vi "NR_LDPC_Decode_opti.vi"(0 "appended path":path, 1 "Zc":dbl, 2 "LDPC_base_graph":dbl, 5 "C":dbl, 9 "cdblkseg_data":dbl[][](array[numeric]), 11 "dermdata":dbl[][](array[numeric]), 12 "EN_LDPC":dbl, 14 "error in (no error)":errorcluster caption="错误输入（无错误）") -> (3 "deldpccode":dbl[][](array[numeric]), 15 "error IO":errorcluster)   [LabVIEW 2015]
panel:
  in  "H":dbl[][](array[numeric])
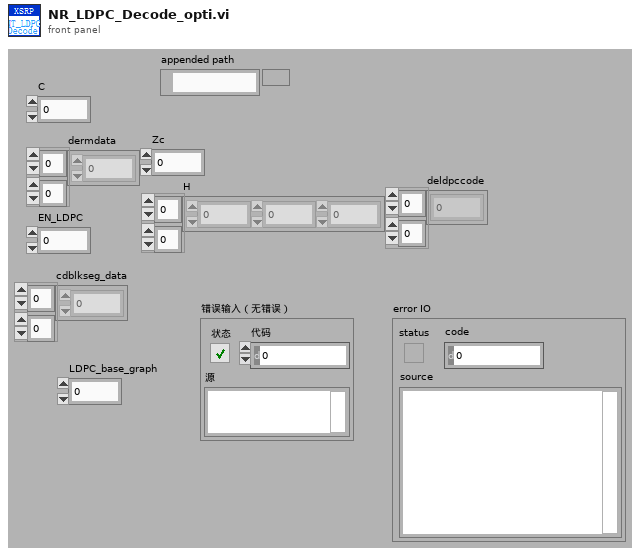
[diagram p1: front panel]
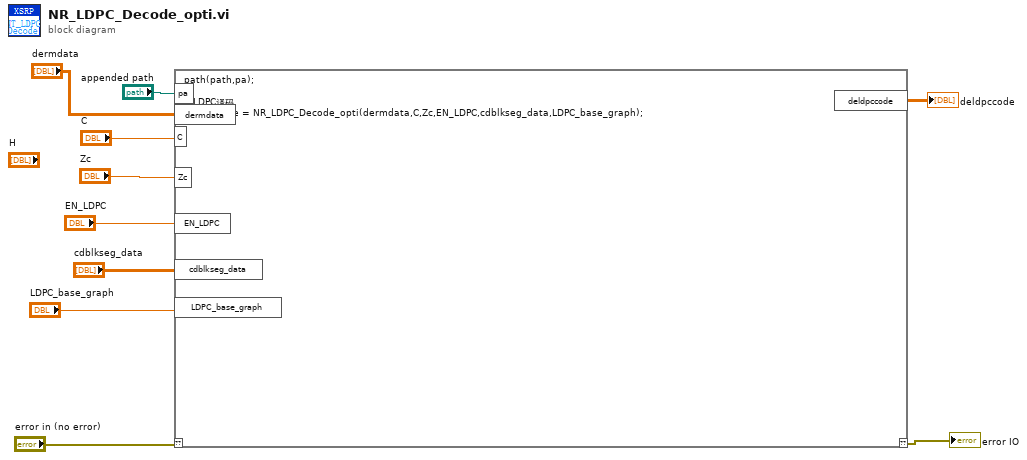
[diagram p0: block diagram]
diagram:
  n1 = script code="path(path,pa);\n\n%LDPC译码\ndeldpccode = NR_LDPC_Decode_opti(dermdata,C,Zc,EN_LDPC,cdblkseg_data,LDPC_base_graph);"("??"="error in (no error)", "pa"="appended path", "dermdata"="dermdata", "C"="C", "Zc"="Zc", "EN_LDPC"="EN_LDPC", "cdblkseg_data"="cdblkseg_data", "LDPC_base_graph"="LDPC_base_graph") -> ("??"=→"error IO":errorcluster, "deldpccode"=→"deldpccode":dbl[][])
